vi "LWXPS_GPIOAnalogConfigurationSet.vi"(6 "LabVIEW error IN":errorcluster, 7 "DAC5 8 Configuration":u32, 8 "DAC1 4 Configuration":u32, 9 "XPS Reference IN":refnum<k24>) -> (0 "LabVIEW error OUT":errorcluster, 1 "XPS Error String":string, 2 "Returned error code":i32, 3 "XPS Reference OUT":refnum<k24>)   [LabVIEW 2014]
uses:
  D:/XPSQ8_LabView_Library/Development/Source/Dll/Newport.XPS.CommandInterface.dll
  Dll/Newport.XPS.CommandInterface.dll
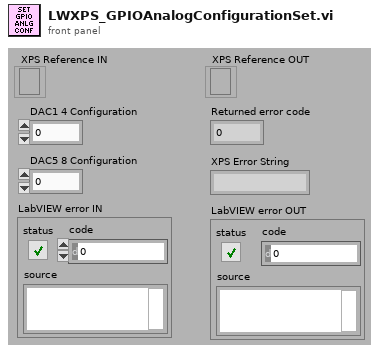
[diagram p1: front panel]
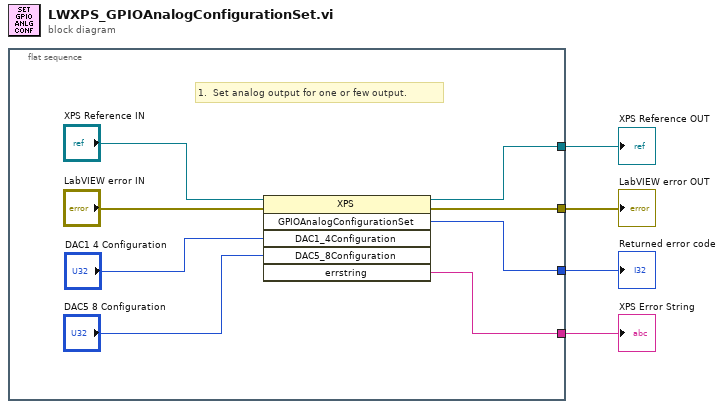
[diagram p0: block diagram]
diagram:
  n1 = flat-sequence {
    tunnel: [w8] -> w4
    tunnel: [w10] -> w3
    tunnel: [w11] -> w2
    tunnel: [w7] -> w1
    frame #0 {
      # "1.  Set analog output for one or few output."
      n2 = invoke class="XPS" method="GPIOAnalogConfigurationSet"(reference="XPS Reference IN", error in="LabVIEW error IN", "DAC1_4Configuration"="DAC1 4 Configuration", "DAC5_8Configuration"="DAC5 8 Configuration") -> (reference out=w8:refnum<k24>, error out=w10:errorcluster, "GPIOAnalogConfigurationSet"=w11:i32, "errstring"=w7:string)  [unwired: 2 in, 2 out]
    }
  }
  "XPS Reference OUT" <- w4
  "LabVIEW error OUT" <- w3
  "Returned error code" <- w2
  "XPS Error String" <- w1
